vi "15.扫描引擎同步 (Host).vi"() -> ()   [LabVIEW 2019]
uses:
  <vilib>/Platform/TimedLoop/XDataNode/timing_clust.ctl
  <vilib>/Platform/TimedLoop/XDataNode/nitl_modes.ctl
  <vilib>/Platform/TimedLoop/XDataNode/wakeup.ctl
  <vilib>/Platform/TimedLoop/XDataNode/loadnilvce.vi
  <vilib>/FPGAPlugInAG/ELVIS III/niLvFpga_Open_ELVIS III.vi
  <vilib>/rvi/interface/common/dynamic/niFpgaDynamicAddResources.vi
  <vilib>/Utility/error.llb/Error Cluster From Error Code.vi
  <vilib>/rvi/errors/niLvFpgaAdjustHostInterfaceError.vi
  <vilib>/FPGAPlugInAG/Dynamic/niLvFpga_Close_Dynamic.vi
  <vilib>/Platform/TimedLoop/XDataNode/XDataNode.xnode
  <vilib>/rvi/interface/nirviOpenFPGA/nirviOpenFPGA.xnode
  <vilib>/rvi/interface/nirviReadWriteControl/nirviReadWriteControl.xnode
  <vilib>/rvi/interface/nirviCloseFPGA/nirviCloseFPGA.xnode
  <vilib>/Platform/TimedLoop/XDataNode/XDNodeRunTimeDep.lvlib
  NiFpgaLv.dll
  <vilib>/rvi/interface/Simulation/niFpgaSimulationCallBeginRW.vi
panel:
  out "error out":errorcluster
  out "Digital Waveform Data from FPGA":i16(graph)
  out "Missed Scan Clock Falling Edge on FPGA":bool
  in  "stop":bool
  out "Host Loop Finished Late? [i-1]":bool
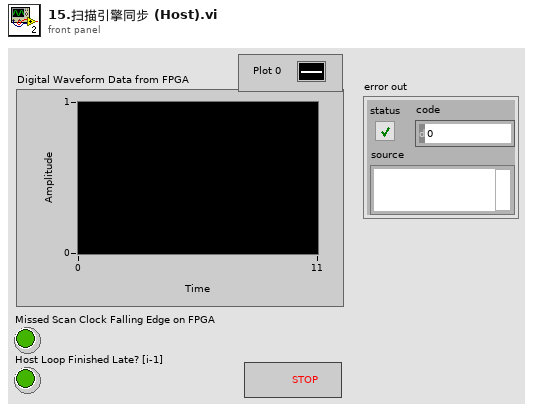
[diagram p1: front panel]
types:
  T1 = typedef "XDNodeRunTimeDep.lvlib/timing_clust.ctl" = cluster{"Expected End [f-1]":u64, "Actual End [f-1]":u64, "Finished Late? [f-1]":bool, "Expected End [i-1]":u64, "Actual End [i-1]":u64, "Finished Late? [i-1]":bool, "Expected Start [i]":u64, "Actual Start [i]":u64, "Expected Start [f]":u64, "Actual Start [f]":u64, "Source Name":string, "Structure Name":string, "Period":i64, "Deadline":i64, "Offset":i64, "Start":i64, "Priority":i32, "Timeout":i32, "Mode":T2, "Wakeup Reason":T3, "Error":errorcluster, "Source Type":string, "Secondary Source Type":string, "Global End Time":u64, "Global Start Time":u64, "Frame Duration":u64, "Iteration Duration":u64, "Assigned CPU":i32, "I/O Scan Engine Mode":u32}
  T2 = typedef "XDNodeRunTimeDep.lvlib/nitl_modes.ctl" = enum32{"No Change", "Process missed periods, maintain original phase", "Discard missed periods, maintain original phase", "Process missed periods, ignore original phase", "Discard missed periods, ignore original phase"}
  T3 = typedef "XDNodeRunTimeDep.lvlib/wakeup.ctl" = enum32{"Normal", "Aborted", "Asynchronous wakeup", "Timing source error", "Timed loop error", "Timeout"}
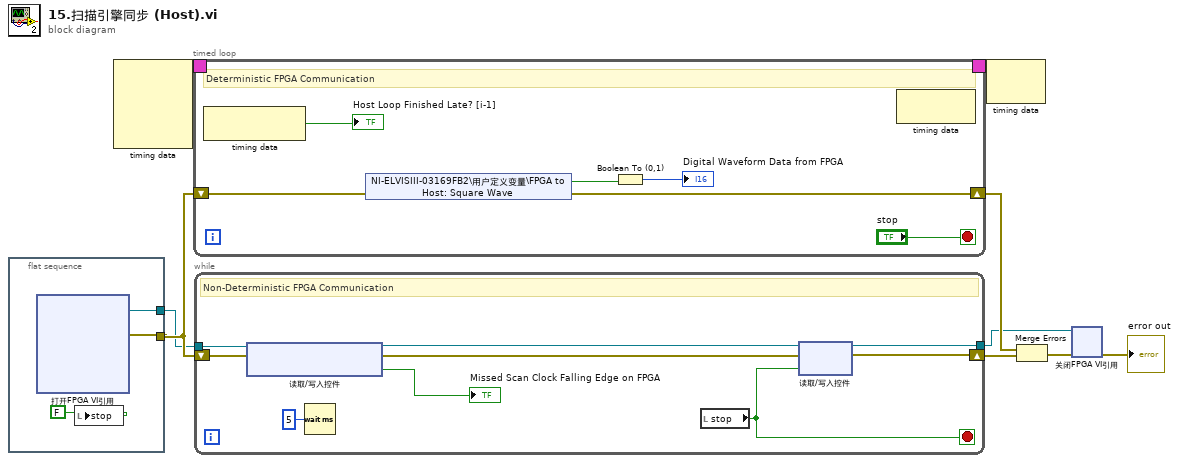
[diagram p0: block diagram]
diagram:
  n1 = flat-sequence {
    tunnel: [w12] -> w7
    tunnel: [w10] -> w6
    frame #0 {
      n2 = xnode "打开FPGA VI引用"() -> ("FPGA VI引用输出"=w10:refnum<k20>, "错误输出"=w12:errorcluster)  [unwired: 2 in]
      n3 = local write "stop"(FALSE) -> ()
    }
  }
  n4 = node-c288() -> (w9:T1)  [unwired: 4 in]
  n5 = timed-loop "定时循环" {
    timing: w9 -> [_]
    timing-out: [_] -> w8
    shift-right: [w13] -> w4
    shift-left: w7 -> [w17]
    stop <- "stop" stop-if-true
    # "Deterministic FPGA Communication"
    n6 = node-c288() -> (→"Host Loop Finished Late? [i-1]":bool)  [unwired: 1 in]
    n7 = shared-variable "NI-ELVISIII-03169FB2\\用户定义变量\\FPGA to Host: Square Wave"(error in=w17) -> (w15:bool, error out=w13:errorcluster)
    n8 = Boolean To (0,1)(Boolean=w15) -> (0, 1=→"Digital Waveform Data from FPGA":i16)
    n9 = node-c288() -> ()  [unwired: 1 in, 1 out]
  }
  n10 = while "While循环" {
    shift-right: [w25] -> w5
    shift-left: w7 -> [w30]
    tunnel: w6 -> [w29]
    tunnel: [w24] -> w2
    stop <- w23 stop-if-true
    # "Non-Deterministic FPGA Communication"
    n11 = xnode "读取/写入控件"("FPGA VI引用输入"=w29, "错误输入"=w30) -> ("FPGA VI引用输出"=w26:refnum<k20>, "错误输出"=w27:errorcluster, "Missed Falling Edge"=→"Missed Scan Clock Falling Edge on FPGA":bool)
    n12 = Wait (ms)(milliseconds to wait=u32 5) -> ()  [unwired: 1 out]
    n13 = local read "stop"() -> (w23:bool)
    n14 = xnode "读取/写入控件"("FPGA VI引用输入"=w26, "错误输入"=w27, "停止"=w23) -> ("FPGA VI引用输出"=w24:refnum<k20>, "错误输出"=w25:errorcluster)
  }
  n15 = node-c288(w8) -> ()  [unwired: 1 out]
  n16 = Merge Errors(w4, w5) -> (w3:errorcluster)
  n17 = xnode "关闭FPGA VI引用"("FPGA VI引用输入"=w2, "错误输入"=w3) -> ("错误输出"=→"error out":errorcluster)
